vi "GUI_main.vi"(11 "Message Queues":T2) -> (0 "error out":errorcluster)   [LabVIEW 2024]
uses:
  CTRLS/Main Tabs.ctl
  CTRLS/Open Batch Data.ctl
  CTRLS/DM_Data.ctl
  CTRLS/run statistics.ctl
  CTRLS/System settings.ctl
  CTRLS/Batch management Control.ctl
  ARCH/Message Queue/All Message Queues.ctl
  ARCH/Message Queue/Message Cluster.ctl
  CTRLS/Printer Message settings.ctl
  CTRLS/REF.ctl
  <vilib>/Utility/miscctls.llb/LVPointTypeDef.ctl
  CTRLS/GLB_VAR.vi
  ARCH/Message Queue/Message Queue.lvlib
  common/virtual_keyboard_lib/Touch_keyboard.lvlib
panel:
  in  "Logout":bool
  in  "Start Printing":bool
  in  "Stop Printing":bool
  out "Printer status":bool
  out "MSG Cenetr":T1
  in  "Navigation":T3
  in  "Main Tab":T4
  in  "Exit":bool
  in  "Login":bool
  in  "Password":string
  in  "Username":string
  out "BatchData":T5
  out "Serial Data":T6 caption="Camera"
  in  "Ready and Paused Batches":string(combo)
  in  "Batch Managment contol":T7
  in  "BatchData MNG":T5
  in  "Export Rejected serials":bool
  in  "Camera Setup":string(combo)="TEST1"
  in  "System settings":T8={"Machine IP"="", "Camera IP"="192.168.250.5", "Printer IP"="192.168.250.3", "Scanner settings"="", "Server Path"=path "", "Sending Port"=3001, "Recieveing Port"=0}
  in  "Save Settings":bool
  in  "Printer Message Config":T9={"Layout File"="2Dmatrix LOTFY.lbl", "Date Separator"="_", "OCR Font"="", "Variable Data"="20 le", "Date Layout"="[MM-DD-YYYY]"}
  out "Run statistics":T10
  out "Batch statistics":T10
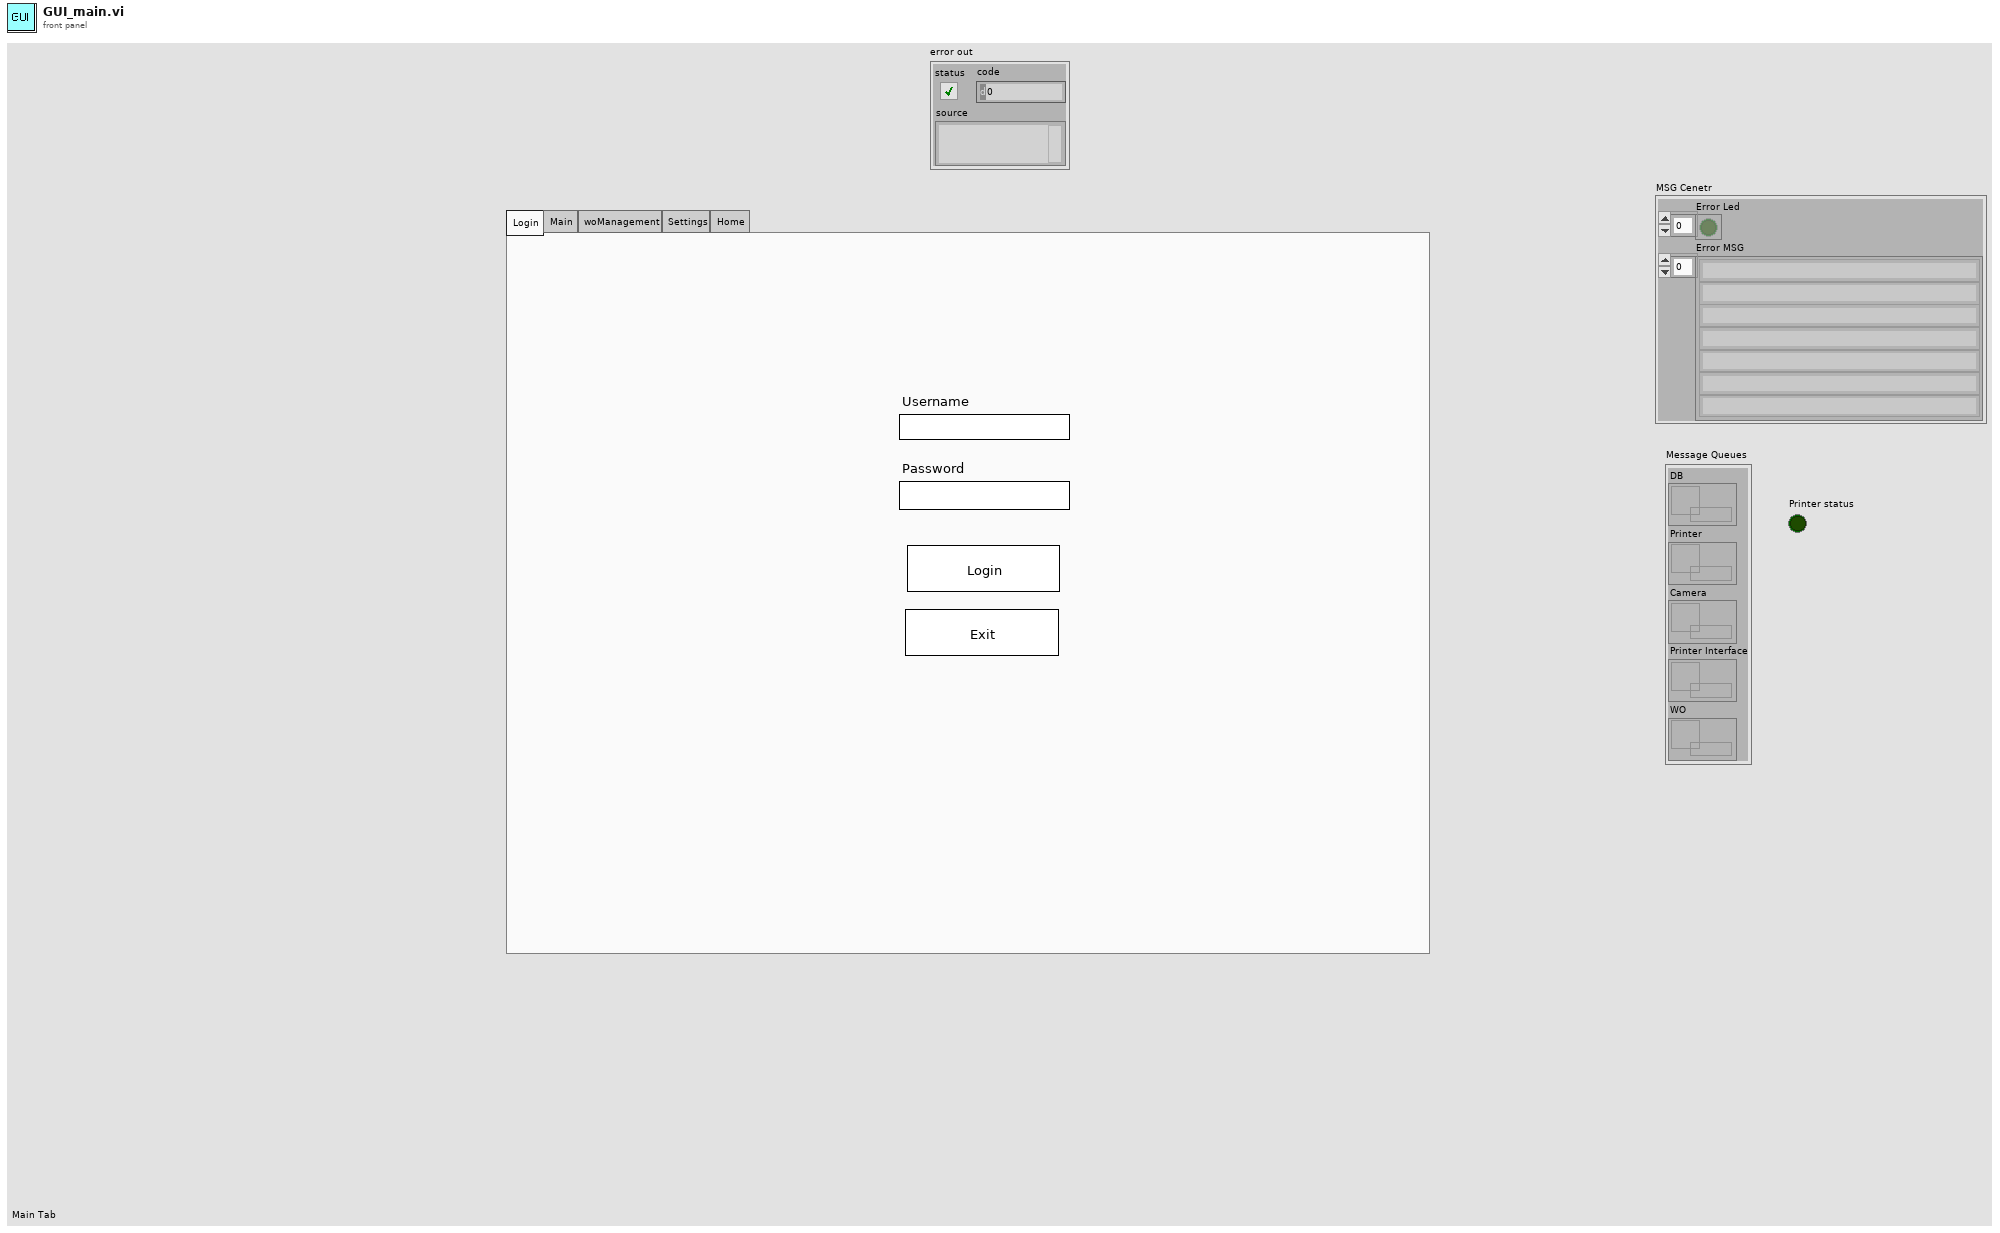
[diagram p1: front panel]
types:
  T1 = cluster{"Error Led":bool[], "Error MSG":string[]}
  T2 = typedef "All Message Queues.ctl" = cluster{"DB":refnum<queue>, "Printer":refnum<queue>, "Camera":refnum<queue>, "Printer Interface":refnum<queue>, "WO":refnum<queue>}
  T3 = cluster{"WO Mng":bool, "Settings":bool, "Main":bool, "Exception Handling":bool, "Home":bool}
  T4 = typedef "Main Tabs.ctl" = enum32{"Login", "Main", "woManagement", "Settings", "Home"}
  T5 = typedef "Open Batch Data.ctl" = cluster{"Batch Name":string, "Batch Number":string, "GTIN":string, "Expiry Date":string, "MFG Date":string}
  T6 = typedef "DM_Data.ctl" = cluster{"2D Code String":string, "Batch Number":string, "GTIN":string, "EXP":string, "Serial":string, "MFG":string}
  T7 = typedef "Batch management Control.ctl" = cluster{"Close Batch":bool, "on hold batch":bool, "Create Batch":bool, "Import Serials":bool, "Generate Serials":bool, "Open batch":bool}
  T8 = typedef "System settings.ctl" = cluster{"Machine IP":string, "Camera IP":string, "Printer IP":string, "Scanner settings":string, "Server Path":path, "Sending Port":u32, "Recieveing Port":u32}
  T9 = typedef "Printer Message settings.ctl" = cluster{"Layout File":string, "Date Separator":string, "OCR Font":string, "Variable Data":string, "Date Layout":string}
  T10 = typedef "run statistics.ctl" = cluster{"Good":dbl, "Bad":dbl, "Good %":dbl, "Bad %":dbl}
  T11 = enum8{"Enabled", "Disabled", "Disabled and Grayed Out"}
  T12 = typedef "LVPointTypeDef.ctl" = cluster{"Horizontal":i16, "Vertical":i16}
  T13 = typedef "REF.ctl" = cluster{"Save Settings":refnum<vi>, "Navigation":refnum<vi>, "Main Tab":refnum<vi>, "Password":refnum<vi>, "BatchData":refnum<vi>, "Serial Data":refnum<vi>, "Username":refnum<vi>, "Stop Printing":refnum<vi>, "Run statistics":refnum<vi>, "System settings":refnum<vi>, "Batch Managment contol":refnum<vi>, "Start Printing":refnum<vi>, "BatchData MNG":refnum<vi>, "MSG Cenetr":refnum<vi>, "Printer status":refnum<vi>, "Printer Message Config":refnum<vi>, "Ready and Paused Batches":refnum<vi>, "Camera Setup":refnum<vi>, "Batch statistics":refnum<vi>, "Logout":refnum<vi>}
  T14 = typedef "Message Queue.lvlib/Message Cluster.ctl" = cluster{"Message":string, "Message Data":variant}
  T15 = typedef "eventvkey.ctl" = enum16{"ASCII", "Enter", "Return", "Shift", "Ctrl", "Alt", "Cmd", "Opt", "Caps", "NumLock", "Clear", "Break", "Up", "Down", "Left", "Right", "Insert", "Delete", "Home", "End", "PageUp", "PageDown", "Escape", "Help", "Pause", "ScrollLock", "F1", "F2", "F3", "F4", "F5", "F6", "F7", "F8", "F9", "F10", "F11", "F12", "F13", "F14", "F15", "F16", "F17", "F18", "F19", "F20", "F21", "F22", "F23", "F24", "Play", "VolumeUp", "VolumeDown", "Mute", "Two Byte Char"}
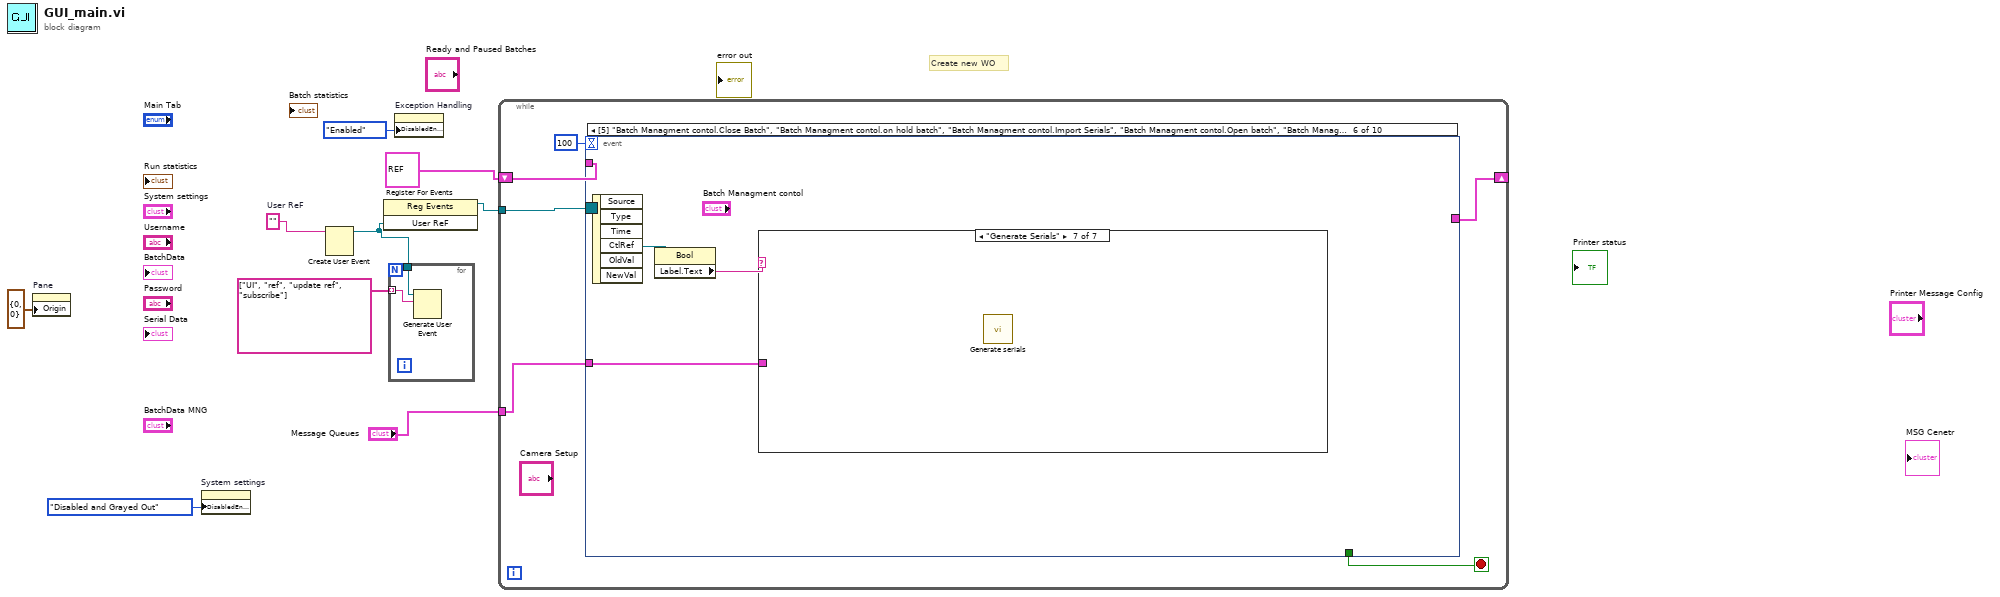
[diagram p0: block diagram]
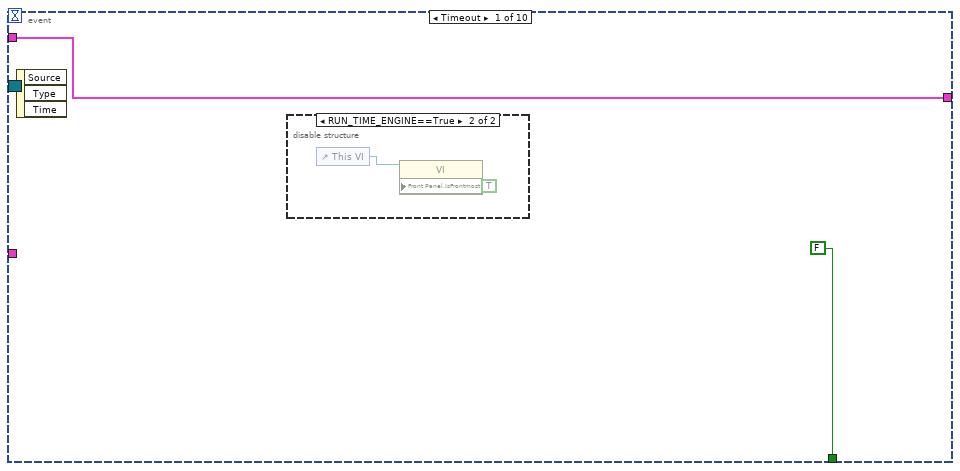
[diagram p2: hidden frame]
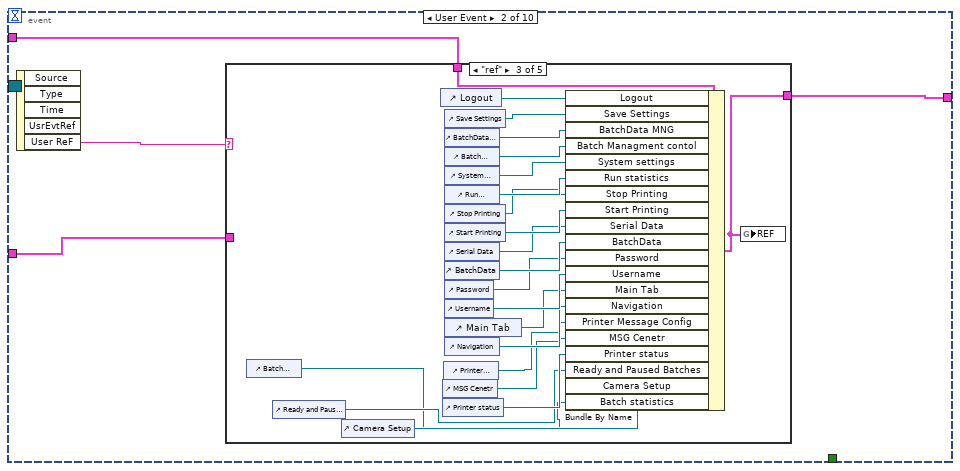
[diagram p4: hidden frame]
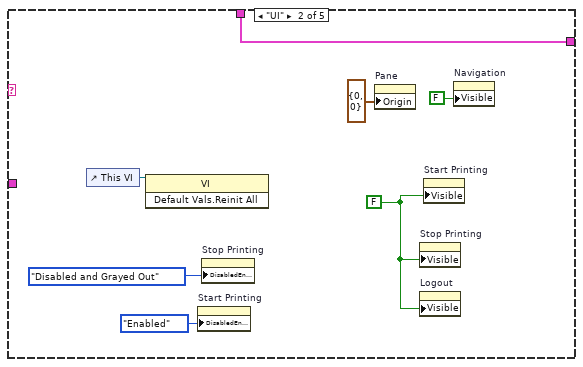
[diagram p6: hidden frame]
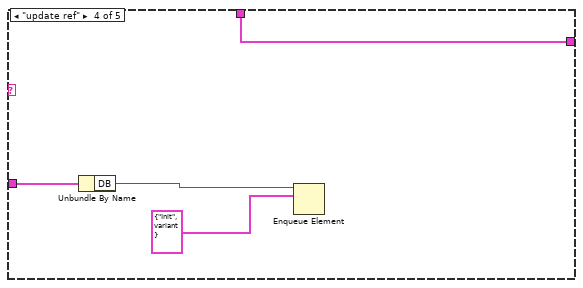
[diagram p7: hidden frame]
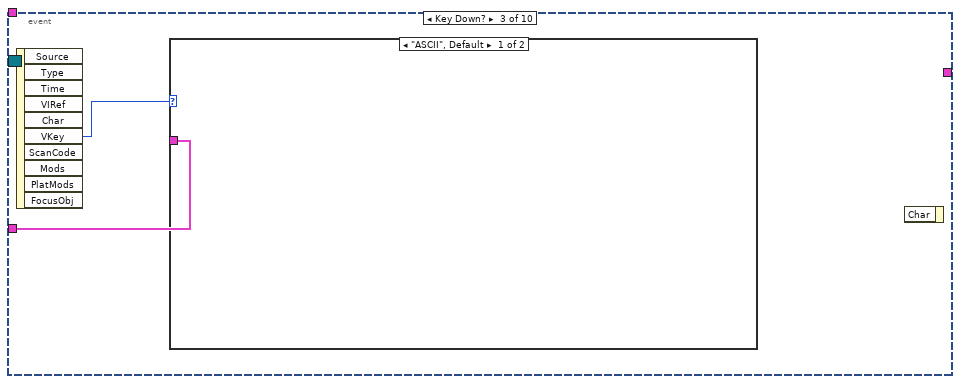
[diagram p9: hidden frame]
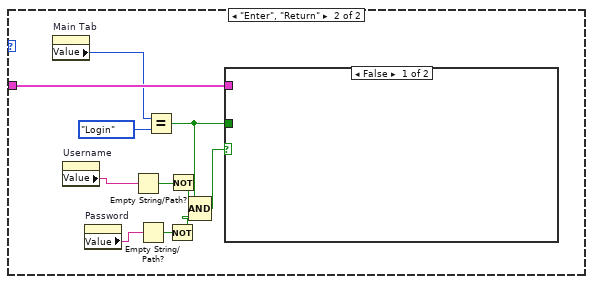
[diagram p10: hidden frame]
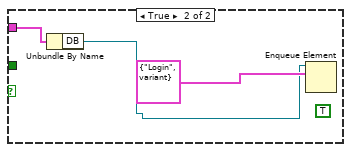
[diagram p11: hidden frame]
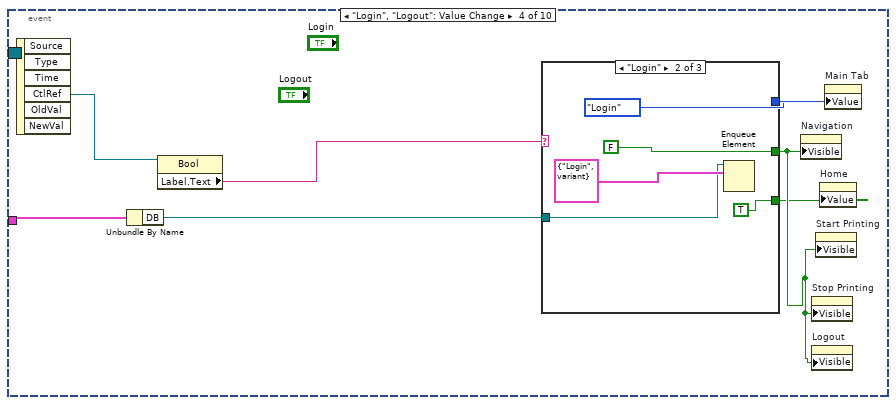
[diagram p12: hidden frame]
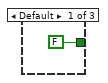
[diagram p13: hidden frame]
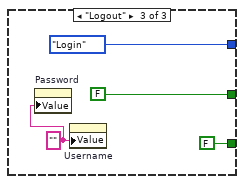
[diagram p14: hidden frame]
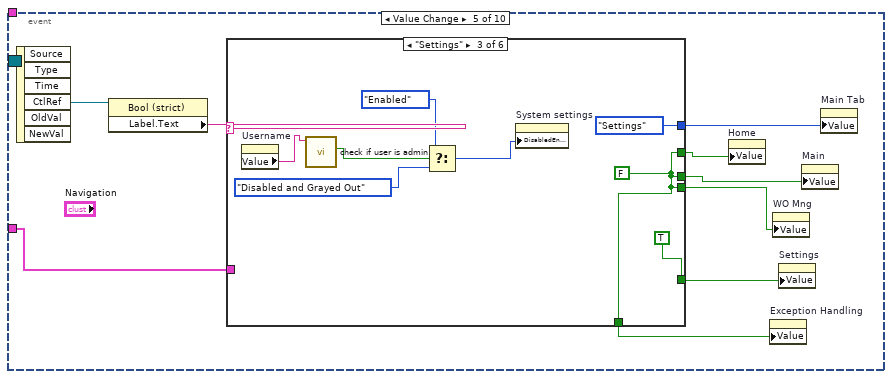
[diagram p15: hidden frame]
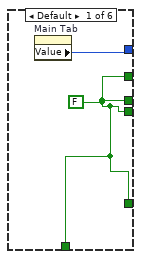
[diagram p16: hidden frame]
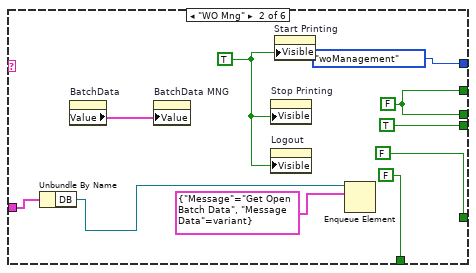
[diagram p17: hidden frame]
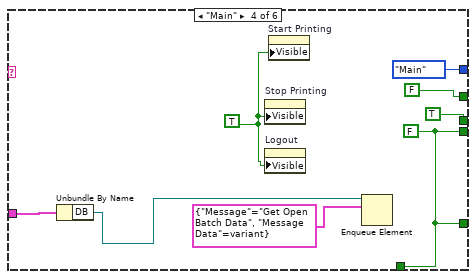
[diagram p18: hidden frame]
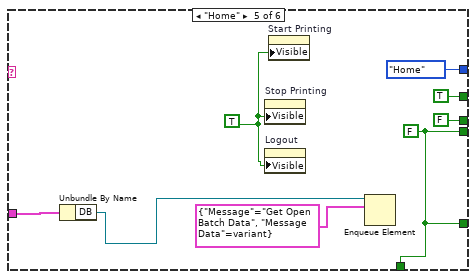
[diagram p19: hidden frame]
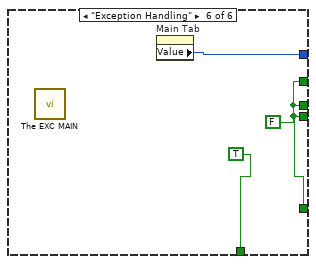
[diagram p20: hidden frame]
diagram:
  w9 = ""  # User ReF
  # "Create new WO"
  n1 = property on="Pane" class="Pane"("Origin"=T12 {"Horizontal"=0, "Vertical"=0}) -> ()  [unwired: 2 in, 2 out]
  n2 = property on="System settings" class="Clust (strict)"("DisabledEnum"=T11."Disabled and Grayed Out" ("Disabled")) -> ()  [unwired: 2 in, 2 out]
  n3 = Create User Event(user event datatype=w9) -> (user event=w6:refnum<user-event>)  [unwired: 1 in, 1 out]
  n4 = register-events(w6) -> (reference out=w8:refnum<event-registration>)  [unwired: 2 in, 1 out]
  n5 = for {
    tunnel: string[] ["UI", "ref", "update ref", "subscribe"] -> [w10] mode=indexing
    tunnel: w6 -> [w11]
    n6 = Generate User Event(user event=w11, event data cluster=w10) -> ()  [unwired: 2 in, 2 out]
  }
  n7 = property on="Exception Handling" class="Bool (strict)"("DisabledEnum"=T11."Enabled" ("Disabled")) -> ()  [unwired: 2 in, 2 out]
  n8 = while {
    tunnel: w8 -> [w16]
    shift-right: [w14] -> _
    shift-left: T13 {"Save Settings"=refnum, "Navigation"=refnum, "Main Tab"=refnum, "Password"=refnum, "BatchData"=refnum, "Serial Data"=refnum, "Username"=refnum, "Stop Printing"=refnum, "Run statistics"=refnum, "System settings"=refnum, "Batch Managment contol"=refnum, "Start Printing"=refnum, "BatchData MNG"=refnum, "MSG Cenetr"=refnum, "Printer status"=refnum, "Printer Message Config"=refnum, "Ready and Paused Batches"=refnum, "Camera Setup"=refnum, "Batch statistics"=refnum, "Logout"=refnum} ("REF") -> [w15]
    tunnel: "Message Queues" -> [w13]
    stop <- w17 stop-if-true
    n9 = event shown="[5] \"Batch Managment contol.Close Batch\", \"Batch Managment contol.on hold batch\", \"Batch Managment contol.Import Serials\", \"Batch Managment contol.Open batch\", \"Batch Managment contol.Create Batch\", \"Batch Managment contol.Generate Serials\": Value Change" {
      selector: w16 -> [_ _ _ _ _ _ _ _ _ _]
      dyn-events: _ -> [_ _ _ _ _ _ _ _ _ _]
      timeout: 100 -> [_ _ _ _ _ _ _ _ _ _]
      tunnel: [FALSE _ _ _ _ _ _ _ _ TRUE] -> w17
      tunnel: w15 -> [w18 w24 _ _ _ _ _ _ _ w272]
      tunnel: [w18 w23 _ _ _ _ _ _ _ w272] -> w14
      tunnel: w13 -> [_ w22 w61 w80 w97 w142 w180 _ w261 w274]
      event Timeout {
        n10 = event-data() -> ()  [unwired: 1 in, 3 out]
        n11 = disable-structure shown="RUN_TIME_ENGINE==True" {
          frame condition #0 (active) {
          }
          frame condition #1 {
            n12 = control-ref of="This VI"() -> (w21:refnum<vi>)
            n13 = property class="VI"(reference=w21, "Front Panel.IsFrontmost"=TRUE ("Front Panel Window:Is Frontmost")) -> ()  [unwired: 1 in, 2 out]
          }
        }
      }
      event User Event {
        n14 = event-data() -> ("User ReF"=w25:string)  [unwired: 1 in, 4 out]
        n15 = case shown="\"ref\"" w25 {
          tunnel: w24 -> [w26 w33 w55 w59 w60]
          tunnel: [w26 w33 w41 w59 w60] -> w23
          tunnel: w22 -> [_ _ _ w56 _]
          frame Default {
          }
          frame "UI" {
            w27 = FALSE ("Visible")
            n16 = control-ref of="This VI"() -> (w30:refnum<vi>)
            n17 = invoke class="VI" method="Default Vals.Reinit All"(reference=w30) -> ()  [unwired: 2 in, 3 out]
            n18 = property on="Start Printing" class="Bool"("DisabledEnum"=T11."Enabled" ("Disabled")) -> ()  [unwired: 2 in, 2 out]
            n19 = property on="Stop Printing" class="Bool"("DisabledEnum"=T11."Disabled and Grayed Out" ("Disabled")) -> ()  [unwired: 2 in, 2 out]
            n20 = property on="Pane" class="Pane"("Origin"=T12 {"Horizontal"=0, "Vertical"=0}) -> ()  [unwired: 2 in, 2 out]
            n21 = property on="Stop Printing" class="Bool"("Visible"=w27) -> ()  [unwired: 2 in, 2 out]
            n22 = property on="Logout" class="Bool"("Visible"=w27) -> ()  [unwired: 2 in, 2 out]
            n23 = property on="Start Printing" class="Bool"("Visible"=w27) -> ()  [unwired: 2 in, 2 out]
            n24 = property on="Navigation" class="Clust (strict)"("Visible"=FALSE) -> ()  [unwired: 2 in, 2 out]
          }
          frame "ref" {
            n25 = control-ref of="Batch statistics"() -> (w35:refnum<vi>)
            n26 = control-ref of="Ready and Paused Batches"() -> (w37:refnum<vi>)
            n27 = control-ref of="Camera Setup"() -> (w36:refnum<vi>)
            n28 = control-ref of="Logout"() -> (w34:refnum<vi>)
            n29 = control-ref of="MSG Cenetr"() -> (w40:refnum<vi>)
            n30 = control-ref of="Printer status"() -> (w39:refnum<vi>)
            n31 = control-ref of="Printer Message Config"() -> (w38:refnum<vi>)
            n32 = control-ref of="Save Settings"() -> (w54:refnum<vi>)
            n33 = control-ref of="BatchData MNG"() -> (w53:refnum<vi>)
            n34 = control-ref of="Batch Managment contol"() -> (w52:refnum<vi>)
            n35 = control-ref of="System settings"() -> (w51:refnum<vi>)
            n36 = control-ref of="Run statistics"() -> (w50:refnum<vi>)
            n37 = control-ref of="Stop Printing"() -> (w49:refnum<vi>)
            n38 = control-ref of="Start Printing"() -> (w48:refnum<vi>)
            n39 = control-ref of="Serial Data"() -> (w47:refnum<vi>)
            n40 = control-ref of="BatchData"() -> (w46:refnum<vi>)
            n41 = control-ref of="Password"() -> (w45:refnum<vi>)
            n42 = control-ref of="Username"() -> (w44:refnum<vi>)
            n43 = control-ref of="Main Tab"() -> (w43:refnum<vi>)
            n44 = control-ref of="Navigation"() -> (w42:refnum<vi>)
            n45 = Bundle By Name(cluster=w55, "Logout"=w34, "Save Settings"=w54, "BatchData MNG"=w53, "Batch Managment contol"=w52, "System settings"=w51, "Run statistics"=w50, "Stop Printing"=w49, "Start Printing"=w48, "Serial Data"=w47, "BatchData"=w46, "Password"=w45, "Username"=w44, "Main Tab"=w43, "Navigation"=w42, "Printer Message Config"=w38, "MSG Cenetr"=w40, "Printer status"=w39, "Ready and Paused Batches"=w37, "Camera Setup"=w36, "Batch statistics"=w35) -> (w41:T13)
            n46 = global write "GLB_VAR.vi" "REF"(w41) -> ()
          }
          frame "update ref" {
            n47 = Unbundle By Name(w56) -> ("DB"=w57:refnum<queue>)
            n48 = Enqueue Element(queue=w57, element=T14 {"Message"="Init", "Message Data"=variant}) -> ()  [unwired: 2 in, 3 out]
          }
          frame "subscribe" {
          }
        }
      }
      event Key Down? {
        n49 = event-data() -> ("VKey"=w62:T15)  [unwired: 1 in, 9 out]
        n50 = case shown="\"ASCII\", Default" w62 {
          tunnel: w61 -> [_ w66]
          frame "ASCII", Default {
          }
          frame "Enter", "Return" {
            n51 = property on="Main Tab" class="TabCtl (strict)"() -> ("Value"=w65:T4)  [unwired: 2 in, 2 out]
            n52 = property on="Username" class="Str"() -> ("Value"=w64:string)  [unwired: 2 in, 2 out]
            n53 = property on="Password" class="Str"() -> ("Value"=w63:string)  [unwired: 2 in, 2 out]
            n54 = Empty String/Path?(string/path=w64) -> (empty?=w72:bool)
            n55 = Empty String/Path?(string/path=w63) -> (empty?=w71:bool)
            n56 = Equal?(x=w65, y=Main_Tabs."Login") -> (x = y?=w70:bool)
            n57 = Not(x=w71) -> (.not. x?=w68:bool)
            n58 = Not(x=w72) -> (.not. x?=w69:bool)
            n59 = Compound Arithmetic op=AND(w70, w69, w68) -> (w67:bool)
            n60 = case shown="False" w67 {
              tunnel: w70 -> [_ _]
              tunnel: w66 -> [_ w74]
              frame False {
              }
              frame True {
                (unwired) TRUE
                n61 = Unbundle By Name(w74) -> ("DB"=w75:refnum<queue>)
                n62 = Enqueue Element(queue=w75, element=T14 {"Message"="Login", "Message Data"=variant}) -> ()  [unwired: 2 in, 3 out]
              }
            }
          }
        }
        n63 = event-data() -> ()  [unwired: 2 in, 1 out]
      }
      event "Login", "Logout": Value Change {
        n64 = event-data() -> ("CtlRef"=w82:refnum<vi>)  [unwired: 1 in, 5 out]
        n65 = Unbundle By Name(w80) -> ("DB"=w79:refnum<queue>)
        n66 = property class="Bool"(reference=w82) -> ("Label.Text"=w81:string)  [unwired: 1 in, 2 out]
        n67 = case shown="\"Login\"" w81 {
          tunnel: [_ Main_Tabs."Login" ("Main Tab") Main_Tabs."Login" ("Main Tab")] -> w83
          tunnel: [_ FALSE ("Visible") FALSE ("Visible")] -> w78
          tunnel: w79 -> [_ w86 _]
          tunnel: [FALSE TRUE FALSE] -> w77
          frame Default {
          }
          frame "Login" {
            n68 = Enqueue Element(queue=w86, element=T14 {"Message"="Login", "Message Data"=variant}) -> ()  [unwired: 2 in, 3 out]
          }
          frame "Logout" {
            w90 = "" ("Username")
            n69 = property on="Password" class="Str"("Value"=w90) -> ()  [unwired: 2 in, 2 out]
            n70 = property on="Username" class="Str"("Value"=w90) -> ()  [unwired: 2 in, 2 out]
          }
        }
        n71 = property on="Navigation" class="Clust (strict)"("Visible"=w78) -> ()  [unwired: 2 in, 2 out]
        n72 = property on="Stop Printing" class="Bool"("Visible"=w78) -> ()  [unwired: 2 in, 2 out]
        n73 = property on="Logout" class="Bool"("Visible"=w78) -> ()  [unwired: 2 in, 2 out]
        n74 = property on="Start Printing" class="Bool"("Visible"=w78) -> ()  [unwired: 2 in, 2 out]
        n75 = property on="Home" class="Bool (strict)"("Value"=w77) -> ()  [unwired: 2 in, 2 out]
        n76 = property on="Main Tab" class="TabCtl (strict)"("Value"=w83) -> ()  [unwired: 2 in, 2 out]
      }
      event "Navigation.WO Mng", "Navigation.Settings", "Navigation.Main", "Navigation.Exception Handling", "Navigation.Home": Value Change {
        n77 = event-data() -> ("CtlRef"=w102:refnum<vi>)  [unwired: 1 in, 5 out]
        n78 = property class="Bool (strict)"(reference=w102) -> ("Label.Text"=w101:string)  [unwired: 1 in, 2 out]
        n79 = case shown="\"Settings\"" w101 {
          tunnel: [w104 Main_Tabs."woManagement" ("Main Tab") Main_Tabs."Settings" ("Main Tab") Main_Tabs."Main" ("Main Tab") Main_Tabs."Home" ("Main Tab") w141] -> w100
          tunnel: [w103 w105 w115 FALSE TRUE w139] -> w95
          tunnel: [w103 TRUE w115 w129 w137 w139] -> w96
          tunnel: [w103 FALSE TRUE w129 w137 w139] -> w99
          tunnel: [w103 FALSE w115 w129 w137 TRUE] -> w98
          tunnel: w97 -> [_ w106 _ w125 w132 _]
          tunnel: [w103 w105 w115 TRUE FALSE w139] -> w94
          frame Default {
            w103 = FALSE
            n80 = property on="Main Tab" class="TabCtl (strict)"() -> ("Value"=w104:T4)  [unwired: 2 in, 2 out]
          }
          frame "WO Mng" {
            w109 = TRUE ("Visible")
            w105 = FALSE
            n81 = Unbundle By Name(w106) -> ("DB"=w107:refnum<queue>)
            n82 = property on="BatchData" class="Clust (strict)"() -> ("Value"=w113:T5)  [unwired: 2 in, 2 out]
            n83 = property on="BatchData MNG" class="Clust (strict)"("Value"=w113) -> ()  [unwired: 2 in, 2 out]
            n84 = property on="Stop Printing" class="Bool"("Visible"=w109) -> ()  [unwired: 2 in, 2 out]
            n85 = property on="Logout" class="Bool"("Visible"=w109) -> ()  [unwired: 2 in, 2 out]
            n86 = property on="Start Printing" class="Bool"("Visible"=w109) -> ()  [unwired: 2 in, 2 out]
            n87 = Enqueue Element(queue=w107, element=T14 {"Message"="Get Open Batch Data", "Message Data"=variant}) -> ()  [unwired: 2 in, 3 out]
          }
          frame "Settings" {
            w115 = FALSE
            n88 = property on="Username" class="Str"() -> ("Value"=w120:string)  [unwired: 2 in, 2 out]
            n89 = call "check if user is admin.vi"("username"=w120) -> ("user is admin"=w119:bool)  [unwired: 10 in]
            n90 = Select(t=T11."Enabled" ("Disabled"), s=w119, f=T11."Disabled and Grayed Out" ("Disabled")) -> (s? t:f=w116:T11)
            n91 = property on="System settings" class="Clust (strict)"("DisabledEnum"=w116) -> ()  [unwired: 2 in, 2 out]
          }
          frame "Main" {
            w127 = TRUE
            w129 = FALSE
            n92 = Unbundle By Name(w125) -> ("DB"=w124:refnum<queue>)
            n93 = property on="Stop Printing" class="Bool"("Visible"=w127) -> ()  [unwired: 2 in, 2 out]
            n94 = property on="Logout" class="Bool"("Visible"=w127) -> ()  [unwired: 2 in, 2 out]
            n95 = property on="Start Printing" class="Bool"("Visible"=w127) -> ()  [unwired: 2 in, 2 out]
            n96 = Enqueue Element(queue=w124, element=T14 {"Message"="Get Open Batch Data", "Message Data"=variant}) -> ()  [unwired: 2 in, 3 out]
          }
          frame "Home" {
            w135 = TRUE
            w137 = FALSE
            n97 = Unbundle By Name(w132) -> ("DB"=w133:refnum<queue>)
            n98 = property on="Stop Printing" class="Bool"("Visible"=w135) -> ()  [unwired: 2 in, 2 out]
            n99 = property on="Logout" class="Bool"("Visible"=w135) -> ()  [unwired: 2 in, 2 out]
            n100 = property on="Start Printing" class="Bool"("Visible"=w135) -> ()  [unwired: 2 in, 2 out]
            n101 = Enqueue Element(queue=w133, element=T14 {"Message"="Get Open Batch Data", "Message Data"=variant}) -> ()  [unwired: 2 in, 3 out]
          }
          frame "Exception Handling" {
            w139 = FALSE
            n102 = call "The EXC MAIN.vi"() -> ()  [unwired: 12 in]
            n103 = property on="Main Tab" class="TabCtl (strict)"() -> ("Value"=w141:T4)  [unwired: 2 in, 2 out]
          }
        }
        n104 = property on="Home" class="Bool (strict)"("Value"=w95) -> ()  [unwired: 2 in, 2 out]
        n105 = property on="Exception Handling" class="Bool (strict)"("Value"=w98) -> ()  [unwired: 2 in, 2 out]
        n106 = property on="WO Mng" class="Bool (strict)"("Value"=w96) -> ()  [unwired: 2 in, 2 out]
        n107 = property on="Settings" class="Bool (strict)"("Value"=w99) -> ()  [unwired: 2 in, 2 out]
        n108 = property on="Main" class="Bool (strict)"("Value"=w94) -> ()  [unwired: 2 in, 2 out]
        n109 = property on="Main Tab" class="TabCtl (strict)"("Value"=w100) -> ()  [unwired: 2 in, 2 out]
      }
      event Value Change {
        n110 = event-data() -> ("CtlRef"=w144:refnum<vi>)  [unwired: 1 in, 5 out]
        n111 = property class="Bool"(reference=w144) -> ("Label.Text"=w143:string)  [unwired: 1 in, 2 out]
        n112 = case shown="\"Generate Serials\"" w143 {
          tunnel: w142 -> [_ w153 w165 w171 w175 _ _]
          frame Default {
          }
          frame "Close Batch" {
            n113 = property on="BatchData" class="Clust (strict)"() -> ("Value"=w147:T5)  [unwired: 2 in, 2 out]
            n114 = Unbundle By Name(w147) -> ("Batch Name"=w146:string)
            n115 = Format Into String(format string="Do you want to close the batch \"%s\"?" ("Title IN"), w146) -> (resulting string=w145:string)  [unwired: 2 in, 1 out]
            n116 = call "Pop up.vi"("Close Visible"=TRUE, "cancel Text"="No", "OK Boolean Text"="Yes", "Title IN"=w145) -> ("Result"=w149:bool)  [unwired: 6 in, 1 out]
            n117 = case shown="True" w149 {
              tunnel: w153 -> [_ w154]
              frame False {
              }
              frame True {
                n118 = Unbundle By Name(w154) -> ("DB"=w156:refnum<queue>)
                n119 = Enqueue Element(queue=w156, element=T14 {"Message"="Close Workorder", "Message Data"=variant}) -> ()  [unwired: 2 in, 3 out]
              }
            }
          }
          frame "on hold batch" {
            n120 = property on="BatchData" class="Clust (strict)"() -> ("Value"=w160:T5)  [unwired: 2 in, 2 out]
            n121 = Unbundle By Name(w160) -> ("Batch Name"=w159:string)
            n122 = Format Into String(format string="Do you want to pause the batch \"%s\"?" ("Title IN"), w159) -> (resulting string=w158:string)  [unwired: 2 in, 1 out]
            n123 = call "Pop up.vi"("Close Visible"=TRUE, "cancel Text"="No", "OK Boolean Text"="Yes", "Title IN"=w158) -> ("Result"=w157:bool)  [unwired: 6 in, 1 out]
            n124 = case shown="True" w157 {
              tunnel: w165 -> [_ w166]
              frame False {
              }
              frame True {
                n125 = Unbundle By Name(w166) -> ("DB"=w168:refnum<queue>)
                n126 = Enqueue Element(queue=w168, element=T14 {"Message"="Pause Workorder", "Message Data"=variant}) -> ()  [unwired: 2 in, 3 out]
              }
            }
          }
          frame "Create Batch" {
            n127 = property on="BatchData MNG" class="Clust (strict)"() -> ("Value"=w170:T5)  [unwired: 2 in, 2 out]
            n128 = call "check batch data.vi"("BatchData MNG"=w170) -> ("valid Data?"=w169:bool)  [unwired: 9 in, 1 out]
            n129 = case shown="True" w169 {
              tunnel: w171 -> [_ w172]
              frame False {
              }
              frame True {
                n130 = Unbundle By Name(w172) -> ("DB"=w174:refnum<queue>)
                n131 = Enqueue Element(queue=w174, element=T14 {"Message"="Create new WO", "Message Data"=variant}) -> ()  [unwired: 2 in, 3 out]
              }
            }
          }
          frame "Open batch" {
            n132 = Unbundle By Name(w175) -> ("DB"=w177:refnum<queue>)
            n133 = Enqueue Element(queue=w177, element=T14 {"Message"="Open Workorder", "Message Data"=variant}) -> ()  [unwired: 2 in, 3 out]
          }
          frame "Import Serials" {
            n134 = call "Import Serials Main.vi"() -> ()  [unwired: 12 in]
          }
          frame "Generate Serials" {
            n135 = call "Generate serials.vi"() -> ()  [unwired: 12 in]
          }
        }
      }
      event "Start Printing", "Save Settings", "Stop Printing": Value Change {
        n136 = event-data() -> ("CtlRef"=w181:refnum<vi>)  [unwired: 1 in, 5 out]
        n137 = property class="Bool"(reference=w181) -> ("Label.Text"=w179:string)  [unwired: 1 in, 2 out]
        n138 = property on="BatchData" class="Clust (strict)"() -> ("Value"=w178:T5)  [unwired: 2 in, 2 out]
        n139 = case shown="\"Save Settings\"" w179 {
          tunnel: w180 -> [_ w188 w192 w199]
          tunnel: w178 -> [_ w187 _ _]
          frame Default {
          }
          frame "Start Printing" {
            n140 = Unbundle By Name(w187) -> ("Batch Number"=w186:string, "GTIN"=w185:string)
            n141 = Unbundle By Name(w188) -> ("DB"=w189:refnum<queue>)
            n142 = Empty String/Path?(string/path=w186) -> (empty?=w184:bool)
            n143 = Empty String/Path?(string/path=w185) -> (empty?=w183:bool)
            n144 = Or(x=w184, y=w183) -> (x .or. y?=w182:bool)
            n145 = case shown="True" w182 {
              tunnel: w189 -> [w191 _]
              frame False {
                n146 = Enqueue Element(queue=w191, element=T14 {"Message"="Start Batch", "Message Data"=variant}) -> ()  [unwired: 2 in, 3 out]
              }
              frame True {
              }
            }
          }
          frame "Stop Printing" {
            n147 = Unbundle By Name(w192) -> ("DB"=w194:refnum<queue>)
            n148 = Enqueue Element(queue=w194, element=T14 {"Message"="Stop Batch", "Message Data"=variant}) -> ()  [unwired: 2 in, 3 out]
          }
          frame "Save Settings" {
            n149 = Unbundle By Name(w199) -> ("Printer Interface"=w198:refnum<queue>, "DB"=w195:refnum<queue>)
            n150 = Enqueue Element(queue=w195, element=T14 {"Message"="Update settings", "Message Data"=variant}) -> ()  [unwired: 2 in, 3 out]
            n151 = Enqueue Element(queue=w198, element=T14 {"Message"="Load Project", "Message Data"=variant}) -> ()  [unwired: 2 in, 3 out]
          }
        }
      }
      event "Username", "Password", "Camera Setup": Mouse Down? {
        n152 = event-data() -> ("CtlRef"=w201:refnum<vi>)  [unwired: 1 in, 7 out]
        n153 = property class="Ctl"(reference=w201) -> ("Label.Text"=w200:string)  [unwired: 1 in, 2 out]
        n154 = case shown="\"Camera Setup\"" w200 {
          frame "False", Default {
          }
          frame "Username" {
            n155 = property on="Username" class="Str"() -> ("Value"=w202:string)  [unwired: 2 in, 2 out]
            n156 = call "HMI Pop Up Alpha KB.vi"("Max Length (70)"=300, "Text"=w202, "String In"=w202) -> ("String Out"=w203:string)  [unwired: 6 in, 2 out]
            n157 = property on="Username" class="Str"("Value"=w203) -> ()  [unwired: 2 in, 2 out]
          }
          frame "Password" {
            n158 = property on="Password" class="Str"() -> ("Value"=w205:string)  [unwired: 2 in, 2 out]
            n159 = call "HMI Pop Up Alpha KB.vi"("Password Display (F)"=TRUE, "Max Length (70)"=300, "Text"=w205, "String In"=w205) -> ("String Out"=w206:string)  [unwired: 5 in, 2 out]
            n160 = property on="Password" class="Str"("Value"=w206) -> ()  [unwired: 2 in, 2 out]
          }
          frame "Batch Name" {
            n161 = property on="Batch Name" class="Str"() -> ("Value"=w209:string)  [unwired: 2 in, 2 out]
            n162 = call "HMI Pop Up Alpha KB.vi"("Password Display (F)"=FALSE, "Max Length (70)"=300, "Text"=w209, "String In"=w209) -> ("String Out"=w210:string)  [unwired: 5 in, 2 out]
            n163 = property on="Batch Name" class="Str"("Value"=w210) -> ()  [unwired: 2 in, 2 out]
          }
          frame "Batch Number" {
            n164 = property on="Batch Number" class="Str"() -> ("Value"=w213:string)  [unwired: 2 in, 2 out]
            n165 = call "HMI Pop Up Alpha KB.vi"("Password Display (F)"=FALSE, "Max Length (70)"=300, "Text"=w213, "String In"=w213) -> ("String Out"=w214:string)  [unwired: 5 in, 2 out]
            n166 = property on="Batch Number" class="Str"("Value"=w214) -> ()  [unwired: 2 in, 2 out]
          }
          frame "GTIN" {
            n167 = property on="GTIN" class="Str"() -> ("Value"=w217:string)  [unwired: 2 in, 2 out]
            n168 = call "HMI Pop Up Num KP.vi"("Password Display (F)"=FALSE, "Max Length (50)"=300 ("Max Length (70)"), "Text"=w217, "String In"=w217) -> ("String Out"=w218:string)  [unwired: 6 in, 1 out]
            n169 = property on="GTIN" class="Str"("Value"=w218) -> ()  [unwired: 2 in, 2 out]
          }
          frame "Expiry Date" {
            (unwired) FALSE ("Password Display (F)")
            n170 = property on="Expiry Date" class="Str"() -> ("Value"=w221:string)  [unwired: 2 in, 2 out]
            n171 = call "HMI Pop Up Alpha KB.vi"("Max Length (70)"=6 ("Max Length (50)"), "Text"=w221, "String In"=w221) -> ("String Out"=w222:string)  [unwired: 6 in, 2 out]
            n172 = property on="Expiry Date" class="Str"("Value"=w222) -> ()  [unwired: 2 in, 2 out]
          }
          frame "MFG Date" {
            (unwired) FALSE ("Password Display (F)")
            n173 = property on="MFG Date" class="Str"() -> ("Value"=w224:string)  [unwired: 2 in, 2 out]
            n174 = call "HMI Pop Up Alpha KB.vi"("Max Length (70)"=6 ("Max Length (50)"), "Text"=w224, "String In"=w224) -> ("String Out"=w225:string)  [unwired: 6 in, 2 out]
            n175 = property on="MFG Date" class="Str"("Value"=w225) -> ()  [unwired: 2 in, 2 out]
          }
          frame "Machine IP" {
            n176 = property on="Machine IP" class="Str"() -> ("Value"=w227:string)  [unwired: 2 in, 2 out]
            n177 = call "HMI Pop Up Alpha KB.vi"("Password Display (F)"=FALSE, "Max Length (70)"=300, "Text"=w227, "String In"=w227) -> ("String Out"=w228:string)  [unwired: 5 in, 2 out]
            n178 = property on="Machine IP" class="Str"("Value"=w228) -> ()  [unwired: 2 in, 2 out]
          }
          frame "Camera IP" {
            (unwired) FALSE ("Password Display (F)")
            n179 = property on="Camera IP" class="Str"() -> ("Value"=w231:string)  [unwired: 2 in, 2 out]
            n180 = call "HMI Pop Up Alpha KB.vi"("Password Display (F)"=FALSE, "Max Length (70)"=300, "Text"=w231, "String In"=w231) -> ("String Out"=w232:string)  [unwired: 5 in, 2 out]
            n181 = property on="Camera IP" class="Str"("Value"=w232) -> ()  [unwired: 2 in, 2 out]
          }
          frame "Printer IP" {
            (unwired) 30 ("Max Length (50)")
            (unwired) FALSE ("Password Display (F)")
            n182 = property on="Printer IP" class="Str"() -> ("Value"=w235:string)  [unwired: 2 in, 2 out]
            n183 = call "HMI Pop Up Alpha KB.vi"("Password Display (F)"=FALSE, "Max Length (70)"=300, "Text"=w235, "String In"=w235) -> ("String Out"=w236:string)  [unwired: 5 in, 2 out]
            n184 = property on="Printer IP" class="Str"("Value"=w236) -> ()  [unwired: 2 in, 2 out]
          }
          frame "Sending Port" {
            (unwired) FALSE ("Password Display (F)")
            n185 = property on="Sending Port" class="DigNum (strict)"() -> ("Value"=w240:u32)  [unwired: 2 in, 2 out]
            n186 = Number To Decimal String(number=w240) -> (decimal integer string=w239:string)  [unwired: 1 in]
            n187 = call "HMI Pop Up Num KP.vi"("Max Length (50)"=30, "Text"=w239, "String In"=w239) -> ("String Out"=w242:string)  [unwired: 7 in, 1 out]
            n188 = Decimal String To Number(string=w242) -> (number=w241:i32)  [unwired: 2 in, 1 out]
            n189 = property on="Sending Port" class="DigNum (strict)"("Value"=w241) -> ()  [unwired: 2 in, 2 out]
          }
          frame "Recieveing Port" {
            (unwired) FALSE ("Password Display (F)")
            n190 = property on="Recieveing Port" class="DigNum (strict)"() -> ("Value"=w245:u32)  [unwired: 2 in, 2 out]
            n191 = Number To Decimal String(number=w245) -> (decimal integer string=w244:string)  [unwired: 1 in]
            n192 = call "HMI Pop Up Num KP.vi"("Max Length (50)"=30, "Text"=w244, "String In"=w244) -> ("String Out"=w247:string)  [unwired: 7 in, 1 out]
            n193 = Decimal String To Number(string=w247) -> (number=w246:i32)  [unwired: 2 in, 1 out]
            n194 = property on="Recieveing Port" class="DigNum (strict)"("Value"=w246) -> ()  [unwired: 2 in, 2 out]
          }
          frame "Scanner settings" {
            n195 = property on="Scanner settings" class="Str"() -> ("Value"=w249:string)  [unwired: 2 in, 2 out]
            n196 = call "HMI Pop Up Alpha KB.vi"("Password Display (F)"=FALSE, "Max Length (70)"=300, "Text"=w249, "String In"=w249) -> ("String Out"=w250:string)  [unwired: 5 in, 2 out]
            n197 = property on="Scanner settings" class="Str"("Value"=w250) -> ()  [unwired: 2 in, 2 out]
          }
          frame "Camera Setup" {
            n198 = property on="Camera Setup" class="CmbBox"() -> ("Value"=w253:string)  [unwired: 2 in, 2 out]
            n199 = call "HMI Pop Up Alpha KB.vi"("Password Display (F)"=FALSE, "Max Length (70)"=300, "Text"=w253, "String In"=w253) -> ("String Out"=w254:string)  [unwired: 5 in, 2 out]
            n200 = property on="Camera Setup" class="CmbBox"("Value"=w254) -> ()  [unwired: 2 in, 2 out]
          }
          frame "Variable Data" {
            n201 = property on="Variable Data" class="Str"() -> ("Value"=w257:string)  [unwired: 2 in, 2 out]
            n202 = call "HMI Pop Up Alpha KB.vi"("Password Display (F)"=FALSE, "Max Length (70)"=300, "Text"=w257, "String In"=w257) -> ("String Out"=w258:string)  [unwired: 5 in, 2 out]
            n203 = property on="Variable Data" class="Str"("Value"=w258) -> ()  [unwired: 2 in, 2 out]
          }
        }
        n204 = event-data() -> ()  [unwired: 2 in, 1 out]
      }
      event "Export Rejected serials": Value Change {
        n205 = event-data() -> ()  [unwired: 1 in, 6 out]
        n206 = property on="BatchData" class="Clust (strict)"() -> ("Value"=w265:T5)  [unwired: 2 in, 2 out]
        n207 = Unbundle By Name(w265) -> ("Batch Number"=w264:string)
        n208 = Empty String/Path?(string/path=w264) -> (empty?=w263:bool)
        n209 = Not(x=w263) -> (.not. x?=w262:bool)
        n210 = case shown="True" w262 {
          tunnel: w261 -> [_ w271]
          frame False {
            n211 = call "Pop up.vi"("Close Visible"=FALSE, "OK Boolean Text"="OK", "Title IN"="No Open Batch") -> ()  [unwired: 7 in, 2 out]
          }
          frame True {
            n212 = Unbundle By Name(w271) -> ("DB"=w270:refnum<queue>)
            n213 = Enqueue Element(queue=w270, element=T14 {"Message"="Export Rejected Serials", "Message Data"=variant}) -> ()  [unwired: 2 in, 3 out]
          }
        }
      }
      event "Exit": Value Change {
        n214 = event-data() -> ()  [unwired: 1 in, 6 out]
        n215 = Cluster To Array(cluster=w274) -> (array=w273:refnum<queue>[])
        n216 = for {
          tunnel: w273 -> [w278] mode=indexing
          n217 = Enqueue Element(queue=w278, element=T14 {"Message"="Exit", "Message Data"=variant}) -> ()  [unwired: 2 in, 3 out]
        }
        n218 = disable-structure shown="RUN_TIME_ENGINE==True" {
          frame condition #0 (active) {
          }
          frame condition #1 {
            n219 = control-ref of="This VI"() -> (w276:refnum<vi>)
            n220 = invoke class="VI" method="FP.Close"(reference=w276) -> ()  [unwired: 2 in, 3 out]
          }
        }
      }
    }
  }
